vi "LED Verification.vi"(8 "Error in":errorcluster caption="Error in (no error)", 11 "String":string) -> (0 "Error out":errorcluster, 3 "Pass":bool)   [LabVIEW 2015, in "Rocom LED Test.lvclass"]
uses:
  Rocom LED Test.lvclass
panel:
  in  "Fail":bool
  in  "Pass":bool=TRUE
  # "LED Verification"
  # "Verify that the LED is"
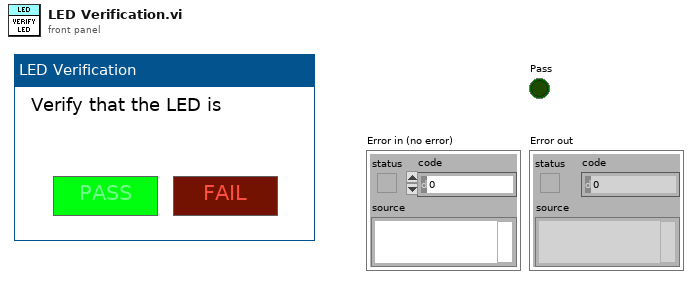
[diagram p1: front panel]
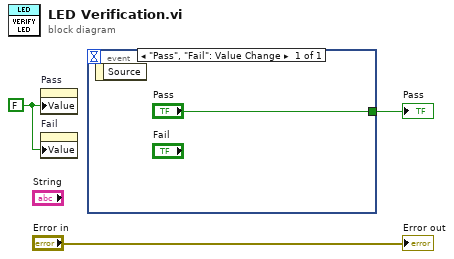
[diagram p0: block diagram]
diagram:
  w1 = FALSE ("LED State")
  n1 = property on="Pass" class="Bool (strict)"("Value"=w1) -> ()  [unwired: 2 in, 2 out]
  n2 = property on="Fail" class="Bool (strict)"("Value"=w1) -> ()  [unwired: 2 in, 2 out]
  n3 = event shown="[0] \"Pass\", \"Fail\": Value Change" {
    selector: _ -> [_]
    dyn-events: _ -> [_]
    timeout: _ -> [_]
    tunnel: ["Pass"] -> w3
    event "Pass", "Fail": Value Change {
      n4 = event-data() -> ()  [unwired: 1 in, 1 out]
    }
  }
  "Pass" <- w3
  "Error out" <- "Error in"
